vi "Build Attribute Tree Data Type.vi"(4 "Show Private?":bool, 5 "Attribute IDs":string[](array[string]), 6 "Item Indent":i32, 7 "Linked List ID":string, 8 "error in (no error)":errorcluster, 9 "Attribute Values":variant[](array[variant]), 10 "Attribute Names":string[](array[string]), 11 "Linked List in":refnum<class "Linked List.lvclass">) -> (0 "error out":errorcluster, 2 "Tree Data Type":T1(array[cluster]), 3 "Linked List out":refnum<class "Linked List.lvclass">)   [LabVIEW 2017, in "Linked Lists.lvlib" / "Linked List.lvclass"]
uses:
  <vilib>/gpm_packages/@cs/linked-list/Source/Linked List/Linked List/Linked List.lvclass
  <vilib>/Utility/Data Type/Get Type Information.vi
  <vilib>/Utility/Data Type/Get Array Information.vi
  <vilib>/Utility/Data Type/Get LabVIEW Class Information.vi
  <vilib>/Utility/Data Type/Get Refnum Information.vi
  <vilib>/gpm_packages/@cs/data-type-serializer/source/Data Type/Data Type.lvclass
  <vilib>/gpm_packages/@cs/variant/Source/VariantExtensions.lvlib
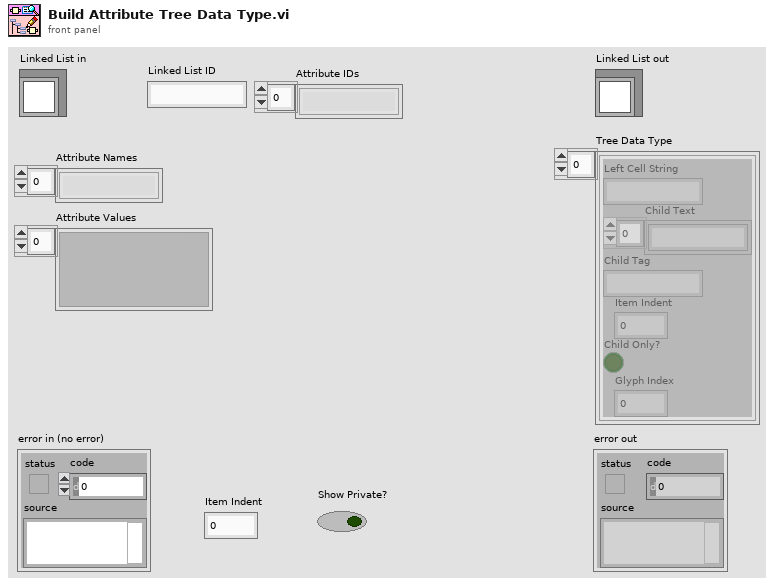
[diagram p1: front panel]
types:
  T1 = cluster{"Left Cell String":string, "Child Text":string[], "Child Tag":string, "Item Indent":i32, "Child Only?":bool, "Glyph Index":i32}[]
  T2 = cluster{"Left Cell String":string, "Child Text":string[], "Child Tag":string, "Item Indent":i32, "Child Only?":bool, "Glyph Index":i32}
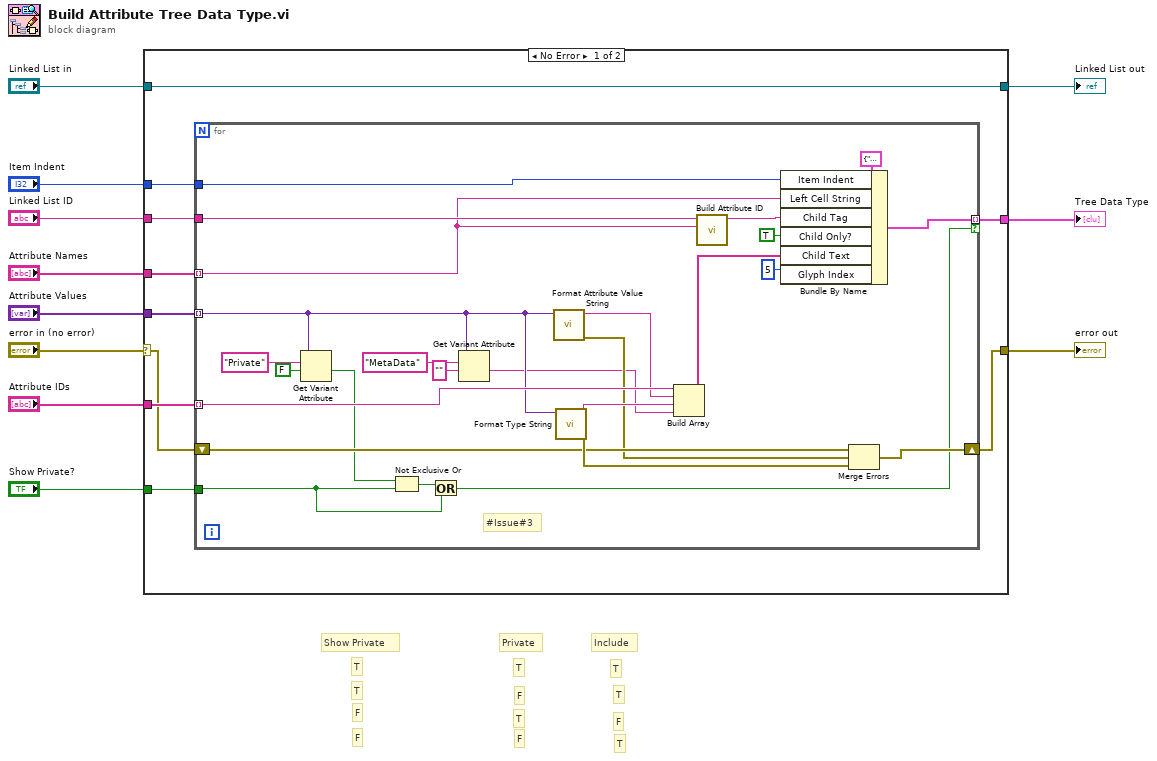
[diagram p0: block diagram]
diagram:
  # "T"
  # "F"
  # "T"
  # "T"
  # "F"
  # "F"
  # "T"
  # "F"
  # "F"
  # "T"
  # "T"
  # "T"
  # "Include"
  # "Private"
  # "Show Private"
  n1 = case shown="No Error" "error in (no error)" {
    selector: "error in (no error)" -> [w12 w48]
    tunnel: "Linked List in" -> [w21 w49]
    tunnel: [w21 w49] -> w9
    tunnel: [w13 w48] -> w8
    tunnel: "Item Indent" -> [w20 _]
    tunnel: "Linked List ID" -> [w19 _]
    tunnel: "Attribute Names" -> [w18 _]
    tunnel: "Attribute Values" -> [w17 _]
    tunnel: "Attribute IDs" -> [w16 _]
    tunnel: "Show Private?" -> [w15 _]
    tunnel: [w14 _] -> w1
    frame No Error {
      n2 = for {
        tunnel: w20 -> [w45]
        tunnel: w19 -> [w44]
        tunnel: w18 -> [w43] mode=indexing
        tunnel: w17 -> [w26] mode=indexing
        tunnel: w16 -> [w41] mode=indexing
        tunnel: w15 -> [w30]
        tunnel: [w39] -> w14 mode=indexing if=w29
        shift-right: [w36] -> w13
        shift-left: w12 -> [w35]
        # "#Issue#3"
        n3 = Get Variant Attribute(Variant=w26, name="Private", default value (empty Variant)=FALSE) -> (value=w32:bool)  [unwired: 1 in, 3 out]
        n4 = Not Exclusive Or(1:w30, 2:w32) -> (0:w31:bool)
        n5 = Or(x=w31, y=w30) -> (x .or. y?=w29:bool)
        n6 = Get Variant Attribute(Variant=w26, name="MetaData", default value (empty Variant)="") -> (value=w23:string)  [unwired: 1 in, 3 out]
        n7 = call <vilib>:"Format Attribute Value String.vi"("Data"=w26) -> ("error out"=w27:errorcluster, "Value as String"=w28:string)  [unwired: 9 in]
        n8 = call <vilib>:"Format Type String.vi"("Data Type"=w26) -> ("error out"=w37:errorcluster, "Type Name"=w38:string)  [unwired: 9 in]
        n9 = Build Array(w41, w28, w38, w23) -> (w40:string[])
        n10 = call <vilib>:"Build Attribute ID.vi"("Attr Name"=w43, "Unique ID"=w44) -> ("Attr ID Out"=w42:string)  [unwired: 9 in]
        n11 = Bundle By Name(cluster=T2 {"Left Cell String"="", "Child Text"=[], "Child Tag"="", "Item Indent"=0, "Child Only?"=FALSE, "Glyph Index"=0} ("Item"), "Item Indent"=w45, "Left Cell String"=w43, "Child Tag"=w42, "Child Only?"=TRUE, "Child Text"=w40, "Glyph Index"=5) -> (w39:T2)
        n12 = Merge Errors(w35, w27, w37) -> (w36:errorcluster)
      }
    }
    frame Error {
    }
  }
  "error out" <- w8
  "Linked List out" <- w9
  "Tree Data Type" <- w1
